vi "librt path.vi"(8 "error in (no error)":errorcluster) -> (0 "error out":errorcluster, 3 "path to librt":path)   [LabVIEW 2013, in "Linux RT IPC.lvlib" / "Shared Memory.lvlib" / "Shared Memory.lvclass"]
doc: "Stores path to standard POSIX library (librt)."
uses:
  Shared Memory.lvclass
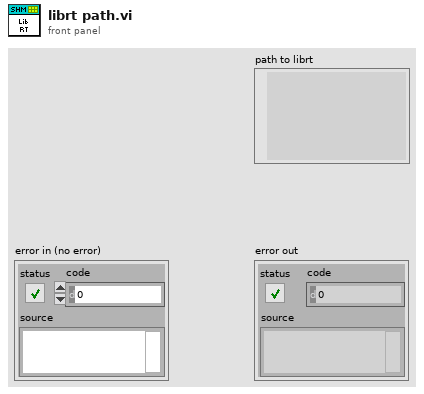
[diagram p1: front panel]
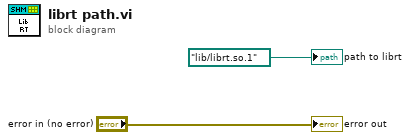
[diagram p0: block diagram]
diagram:
  "error out" <- "error in (no error)"
  "path to librt" <- path "/lib/librt.so.1" ("path to libc")
